vi "Try Measurement Process.vi"() -> ()   [LabVIEW 2015, in "PAS.lvclass"]
uses:
  PAS.lvclass
panel:
  in  "stop":bool
  out "error out":errorcluster
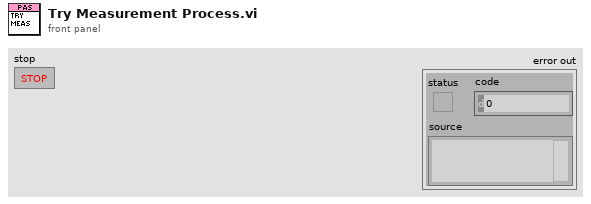
[diagram p1: front panel]
types:
  T1 = typedef "PAS.lvclass/Session Handle.ctl" = refnum<data-value>
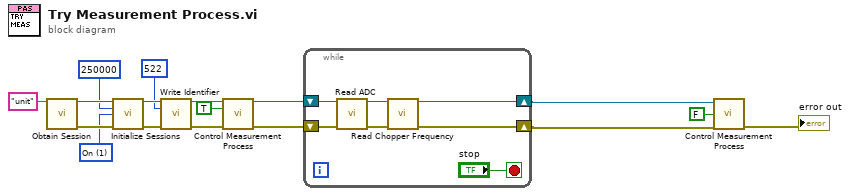
[diagram p0: block diagram]
diagram:
  w13 = u32 1 items=["Off", "On"] ("Termination")
  n1 = call "Obtain Session.vi"("Session  Name ()"="unit") -> ("Session Handle"=w17:T1, "error out"=w16:errorcluster)  [unwired: 13 in]
  n2 = call "Initialize Sessions.vi"("Session Handle in"=w17, "Baud Rate"=u32 250000, "Termination"=w13, "error in (no error)"=w16) -> ("Session Handle Out"=w12:T1, "error out"=w11:errorcluster)  [unwired: 10 in]
  n3 = call "Write Identifier.vi"("Session Handle in"=w12, "identifier"=u16 522, "error in (no error)"=w11) -> ("Session Handle out"=w9:T1, "error out"=w8:errorcluster)  [unwired: 11 in]
  n4 = call "Control Measurement Process.vi"("Session Handle in"=w9, "Start?"=TRUE, "error in (no error)"=w8) -> ("Session Handle out"=w4:T1, "error out"=w3:errorcluster)  [unwired: 9 in, 2 out]
  n5 = while {
    shift-right: [w20] -> w2
    shift-left: w4 -> [w24]
    shift-right: [w19] -> w1
    shift-left: w3 -> [w23]
    stop <- "stop" stop-if-true
    n6 = call "Read ADC.vi"("Session Handle in"=w24, "error in (no error)"=w23) -> ("Session Handle out"=w21:T1, "error out"=w22:errorcluster)  [unwired: 9 in, 3 out]
    n7 = call "Read Chopper Frequency.vi"("Session Handle in"=w21, "error in (no error)"=w22) -> ("Session Handle out"=w20:T1, "error out"=w19:errorcluster)  [unwired: 9 in, 3 out]
  }
  n8 = call "Control Measurement Process.vi"("Session Handle in"=w2, "Start?"=FALSE, "error in (no error)"=w1) -> ("error out"=→"error out":errorcluster)  [unwired: 9 in, 3 out]
